vi "SECoP-addCommand.vi"(6 "description":string, 7 "datainfo":string, 8 "error in (no error)":errorcluster, 10 "command name":string, 11 "DLL path (in)":T1) -> (0 "error out":errorcluster, 3 "DLL path (out)":T1)   [LabVIEW 2023, in "SECoP.lvlib"]
doc: "Call <b>\"SECoP-addCommand.vi\"</b> to create a SECoP command inside the last created SECoP module.\n\n<b>DLL path</b> input and output of cluster from \"SECoP-Initialize.vi\"\n<b>command name</b> name of command\n<b>datainfo</b> data info (data type of command, see SECoP specification)\n<b>description</b> human readable description of this command"
uses:
  SECoP.lvlib
  SECoP-libraries.ctl
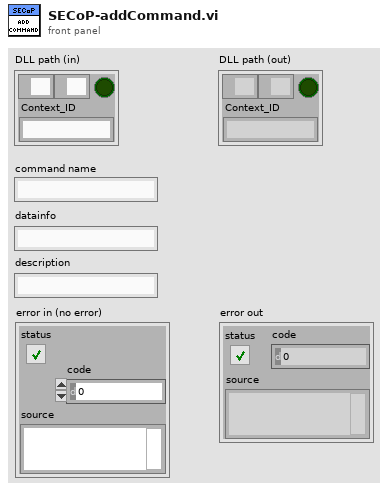
[diagram p1: front panel]
types:
  T1 = typedef "SECoP.lvlib/SECoP-libraries.ctl" = cluster{"serverDLL":path, "variantDLL":path, "cleanup_mode":bool, "Context_ID":string}
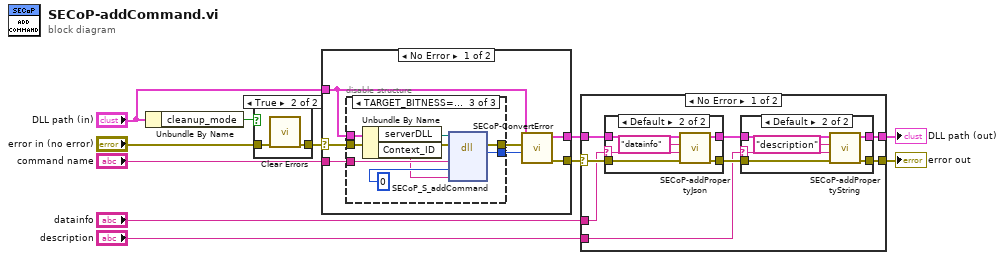
[diagram p0: block diagram]
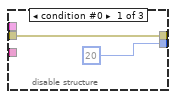
[diagram p6: hidden frame]
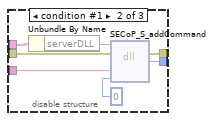
[diagram p7: hidden frame]
diagram:
  n1 = Unbundle By Name("DLL path (in)") -> ("cleanup_mode"=w10:bool)
  n2 = case shown="True" w10 {
    tunnel: "error in (no error)" -> [w12 w14]
    tunnel: [w12 w13] -> w8
    frame False {
    }
    frame True {
      n3 = call <vilib>:"Clear Errors.vi"("error in (no error)"=w14) -> ("error out"=w13:errorcluster)  [unwired: 5 in, 1 out]
    }
  }
  n4 = case shown="No Error" w8 {
    selector: w8 -> [w16 w39]
    tunnel: "DLL path (in)" -> [w15 w40]
    tunnel: [w20 w40] -> w4
    tunnel: [w21 w39] -> w6
    tunnel: "command name" -> [w17 _]
    frame No Error {
      n5 = disable-structure shown="TARGET_BITNESS==64" {
        disable-tunnel: [w23 w30 w38] -> w19
        disable-tunnel: [20 ("return code") w29 w37] -> w18
        disable-tunnel: w17 -> [_ w27 w35]
        disable-tunnel: w16 -> [w23 w26 w34]
        disable-tunnel: w15 -> [_ w25 w33]
        frame condition #0 {
        }
        frame condition #1 {
          n6 = Unbundle By Name(w25) -> ("serverDLL"=w24:path)
          n7 = dll-call lib="Z:/Praktische Aufgaben/SECoP-LabVIEW2015/32bit/SECoP32.dll" fn="SECoP_S_addCommand"(path in=w24, error in=w26, "Name"=w27, "Function pointer"=u32 0) -> (error out=w30:errorcluster, "return type"=w29:i32)  [unwired: 3 in, 1 out]
        }
        frame condition #2 (active) {
          n8 = Unbundle By Name(w33) -> ("serverDLL"=w32:path, "Context_ID"=w31:string)
          n9 = dll-call lib="Z:/Praktische Aufgaben/SECoP-LabVIEW2015/32bit/SECoP32.dll" fn="SECoP_S_addCommand"(path in=w32, error in=w34, "Name"=w35, "Function pointer"=u64 0, "szContextID"=w31) -> (error out=w38:errorcluster, "return type"=w37:i32)  [unwired: 4 in, 1 out]
        }
      }
      n10 = call "SECoP-ConvertError.vi"("return code"=w18, "error in (no error)"=w19, "DLL path (in)"=w15) -> ("error out"=w21:errorcluster, "DLL path (out)"=w20:T1)  [unwired: 7 in]
    }
    frame Error {
    }
  }
  n11 = case shown="No Error" w6 {
    selector: w6 -> [w46 w66]
    tunnel: w4 -> [w47 w65]
    tunnel: [w41 w66] -> w5
    tunnel: [w42 w65] -> w3
    tunnel: "datainfo" -> [w45 _]
    tunnel: "description" -> [w44 _]
    frame No Error {
      n12 = case shown="Default" w45 {
        selector: w45 -> [_ w60]
        tunnel: w47 -> [w58 w64]
        tunnel: w46 -> [w57 w63]
        tunnel: [w57 w62] -> w48
        tunnel: [w58 w61] -> w43
        frame "" {
        }
        frame Default {
          n13 = call "SECoP-addPropertyJson.vi"("error in (no error)"=w63, "property value"=w60, "property name"="datainfo", "DLL path (in)"=w64) -> ("error out"=w62:errorcluster, "DLL path (out)"=w61:T1)  [unwired: 6 in]
        }
      }
      n14 = case shown="Default" w44 {
        selector: w44 -> [_ w52]
        tunnel: w43 -> [w50 w56]
        tunnel: w48 -> [w49 w55]
        tunnel: [w49 w54] -> w41
        tunnel: [w50 w53] -> w42
        frame "" {
        }
        frame Default {
          n15 = call "SECoP-addPropertyString.vi"("error in (no error)"=w55, "property value"=w52, "property name"="description", "DLL path (in)"=w56) -> ("error out"=w54:errorcluster, "DLL path (out)"=w53:T1)  [unwired: 6 in]
        }
      }
    }
    frame Error {
    }
  }
  "DLL path (out)" <- w3
  "error out" <- w5
